vi "Launch Storage Actor.vi"(8 "error in (no error)":errorcluster, 10 "Storage Act":refnum<class "Storage.lvclass">, 11 "HIJ Vision Camera App in":refnum<class "HIJ Vision Camera App.lvclass">) -> (0 "error out":errorcluster, 3 "HIJ Vision Camera App out":refnum<class "HIJ Vision Camera App.lvclass">)   [LabVIEW 2014]
uses:
  <vilib>/ActorFramework/Actor/Actor.lvclass
  HIJ Vision Camera App.lvclass
  Storage/Storage/Storage.lvclass
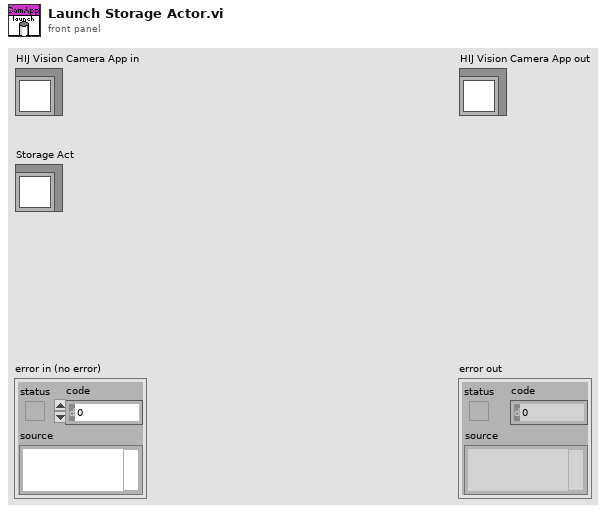
[diagram p1: front panel]
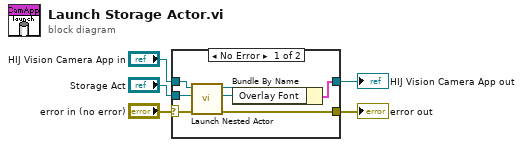
[diagram p0: block diagram]
diagram:
  n1 = case shown="No Error" "error in (no error)" {
    selector: "error in (no error)" -> [w7 w14]
    tunnel: [w6 w14] -> w4
    tunnel: [w9 w13] -> w2
    tunnel: "HIJ Vision Camera App in" -> [w11 w13]
    tunnel: "Storage Act" -> [w10 _]
    frame No Error {
      n2 = call <vilib>:"Launch Nested Actor.vi"("error in (no error)"=w7, "Nested Actor"=w10, "Caller Actor in"=w11) -> ("error out"=w6:errorcluster, "Nested Actor's Enqueuer"=w8:refnum<class "Message Enqueuer.lvclass">, "Caller Actor out"=w12:refnum<class "HIJ Vision Camera App.lvclass">)  [unwired: 6 in]
      n3 = Bundle By Name(cluster=w12, "Overlay Font"=w8) -> (w9:cluster{})
    }
    frame Error {
    }
  }
  "error out" <- w4
  "HIJ Vision Camera App out" <- w2
